vi "vision_targets_to_track_fg.vi"(1 "Input":i32, 2 "Menu (Get)":T1) -> (0 "Output":i32)   [LabVIEW 2012]
uses:
  typedefs/fg_typedef.ctl
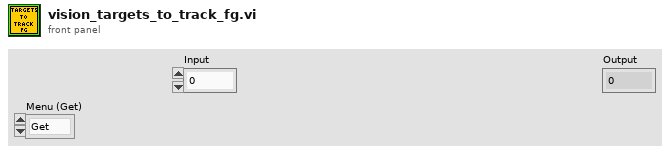
[diagram p1: front panel]
types:
  T1 = typedef "fg_typedef.ctl" = enum16{"Get", "Set"}
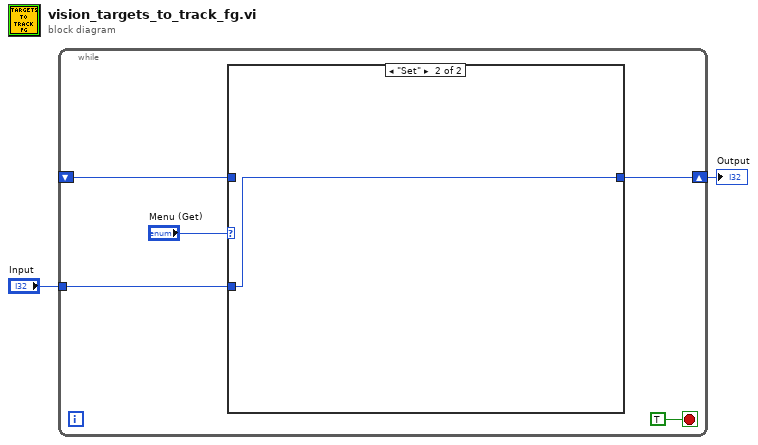
[diagram p0: block diagram]
diagram:
  n1 = while {
    shift-right: [w4] -> w1
    shift-left: _ -> [w5]
    tunnel: "Input" -> [w3]
    stop <- TRUE stop-if-true
    n2 = case shown="\"Set\"" "Menu (Get)" {
      tunnel: w5 -> [w8 _]
      tunnel: [w8 w9] -> w4
      tunnel: w3 -> [_ w9]
      frame "Get", Default {
      }
      frame "Set" {
      }
    }
  }
  "Output" <- w1
